vi "motor_calibration.vi"(0 "NXT/EV3":T2, 1 "Motors":T1=1 items=["Port A", "Port B", "Port C", "Port D"], 4 "Time (1 sec)":sgl=0.57000005 step=0.01) -> (5 "NXT/EV3 2":T2)   [LabVIEW 2013]
uses:
  <vilib>/NXT/Subs/LVHSConnector.ctl
  <vilib>/NXT/LegoClasses/BrickReference/BrickReference.lvclass
  <vilib>/NXT/Block Support/NXT_OutputPort.ctl
  <vilib>/NXT/Dual Mode Library/Waits/Wait_Num.vi
  <vilib>/NXT/NXTIO Xnodes/NXTIONodeSubVIs/NXTStopMotors.vi
  <vilib>/NXT/NXTIO Xnodes/NXTIONodeSubVIs/NXTMoveMotors.vi
  <vilib>/NXT/NXTIO Xnodes/NXTIOXNode/NXTIO.xnode
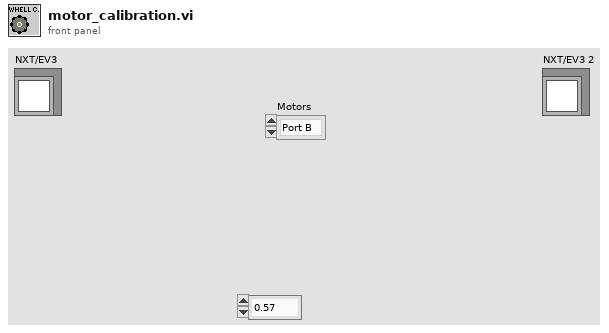
[diagram p1: front panel]
types:
  T1 = typedef "NXT_OutputPort.ctl" = u8
  T2 = typedef "LVHSConnector.ctl" = refnum<class "BrickReference.lvclass">
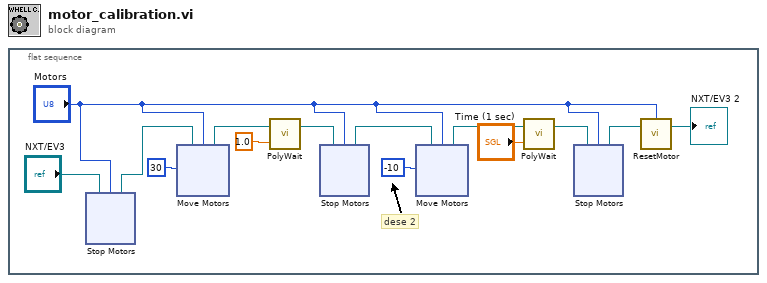
[diagram p0: block diagram]
diagram:
  n1 = flat-sequence {
    frame #0 {
      # "dese 2"
      n2 = xnode "Stop Motors"("Motors"="Motors", "NXT/EV3"="NXT/EV3") -> ("NXT/EV3"=w6:T2)
      n3 = xnode "Move Motors"("Power/Speed 1"=i8 30, "Motors"="Motors", "NXT/EV3"=w6) -> ("NXT/EV3"=w13:T2)
      n4 = call-poly <vilib>:"PolyWait.vi"("Time (1 sec)"=sgl 1.0, "NXT/EV3"=w13) -> ("NXT/EV3"=w11:T2)  [unwired: 2 in]
      n5 = xnode "Stop Motors"("Motors"="Motors", "NXT/EV3"=w11) -> ("NXT/EV3"=w10:T2)
      n6 = xnode "Move Motors"("Power/Speed 1"=i8 -10, "Motors"="Motors", "NXT/EV3"=w10) -> ("NXT/EV3"=w8:T2)
      n7 = call-poly <vilib>:"PolyWait.vi"("Time (1 sec)"="Time (1 sec)", "NXT/EV3"=w8) -> ("NXT/EV3"=w9:T2)  [unwired: 2 in]
      n8 = xnode "Stop Motors"("Motors"="Motors", "NXT/EV3"=w9) -> ("NXT/EV3"=w4:T2)
      n9 = call <vilib>:"ResetMotor.vi"("NXT/EV3"=w4, "Port (All Ports)"="Motors") -> ("NXT/EV3"=→"NXT/EV3 2":T2)  [unwired: 2 in]
    }
  }
